vi "Save Distances.vi"(10 "Cluster":T1, 11 "Process":bool) -> ()   [LabVIEW 2016]
uses:
  <vilib>/Utility/config.llb/Write Key (Double).vi
  <vilib>/Utility/config.llb/NI_LVConfig.lvlib
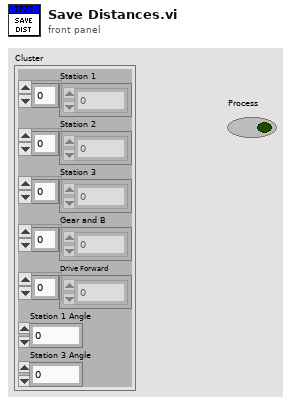
[diagram p1: front panel]
types:
  T1 = cluster{"Station 1":dbl[], "Station 2":dbl[], "Station 3":dbl[], "Gear and B":dbl[], "Drive Forward":dbl[], "Station 1 Angle":dbl, "Station 3 Angle":dbl}
  T2 = typedef "NI_LVConfig.lvlib/Config Data RefNum.ctl" = refnum<k1>
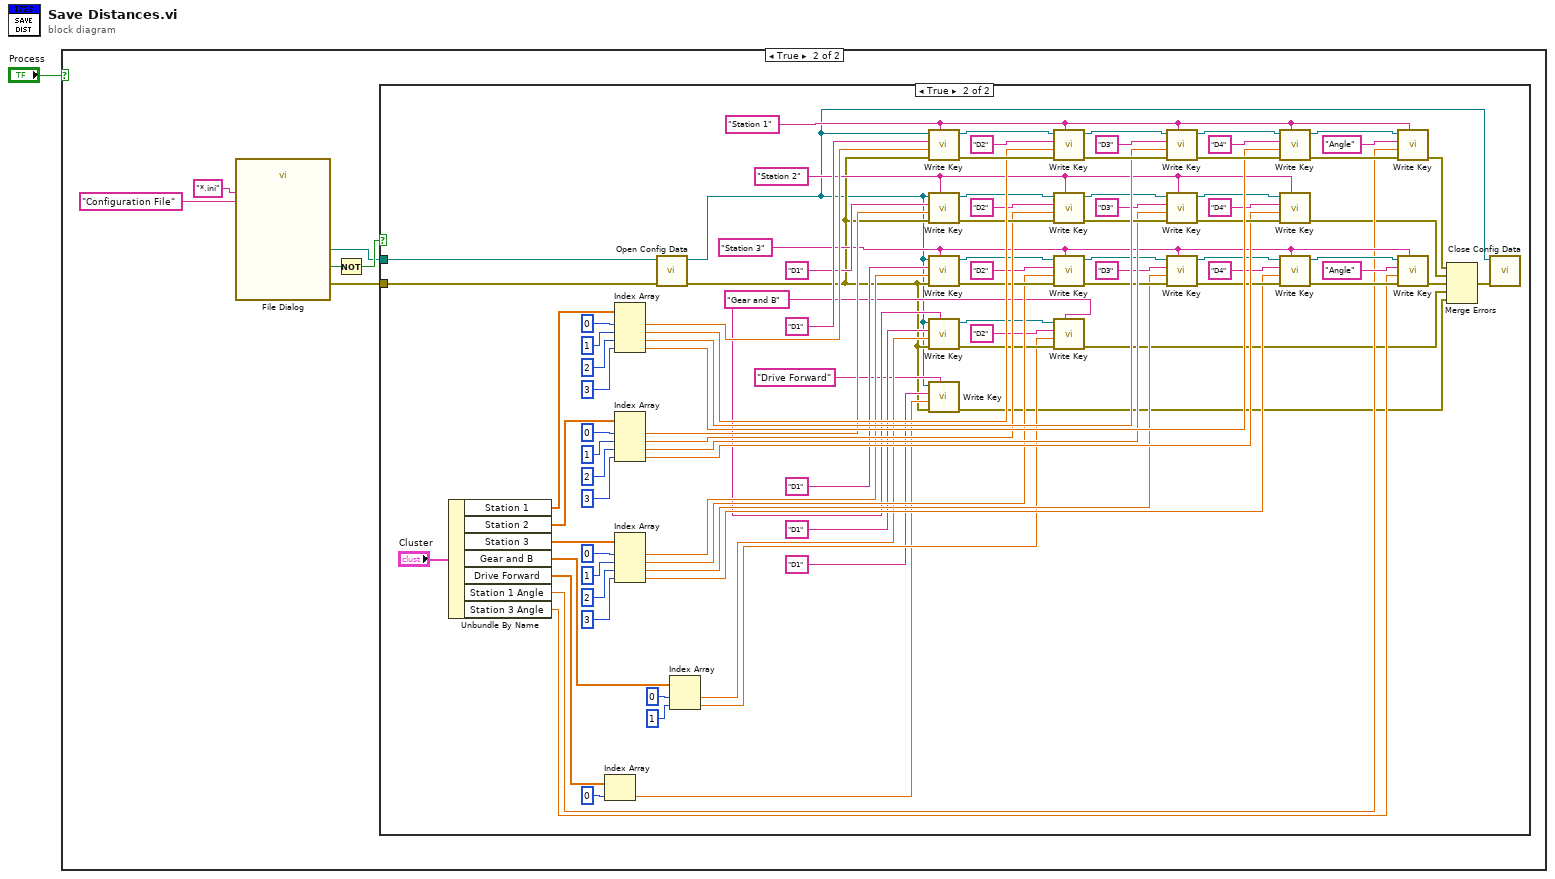
[diagram p0: block diagram]
diagram:
  n1 = case shown="True" "Process" {
    frame False {
    }
    frame True {
      n2 = call "File Dialog"("pattern (all files)"="*.ini", "pattern label"="Configuration File") -> ("selected path"=w5:path, "cancelled"=w7:bool, "error out"=w4:errorcluster)  [unwired: 10 in, 1 out]
      n3 = Not(x=w7) -> (.not. x?=w6:bool)
      n4 = case shown="True" w6 {
        tunnel: w5 -> [_ w100]
        tunnel: w4 -> [_ w99]
        frame False {
        }
        frame True {
          w31 = "Gear and B" ("section")
          w42 = "Station 3" ("section")
          w65 = "Station 2" ("section")
          w76 = "Station 1" ("section")
          n5 = Unbundle By Name("Cluster") -> ("Station 1"=w91:dbl[], "Station 2"=w60:dbl[], "Station 3"=w37:dbl[], "Gear and B"=w24:dbl[], "Drive Forward"=w17:dbl[], "Station 1 Angle"=w19:dbl, "Station 3 Angle"=w32:dbl)
          n6 = Index Array(array=w17, index=0) -> (element=w16:dbl)
          n7 = Index Array(array=w91, index #1=0 ("index"), index #2=1 ("index"), index #3=2 ("index"), index #4=3 ("index")) -> (element #1=w83:dbl, element #2=w82:dbl, element #3=w81:dbl, element #4=w80:dbl)
          n8 = Index Array(array=w60, index #1=0 ("index"), index #2=1 ("index"), index #3=2 ("index"), index #4=3 ("index")) -> (element #1=w59:dbl, element #2=w58:dbl, element #3=w57:dbl, element #4=w56:dbl)
          n9 = Index Array(array=w37, index #1=0 ("index"), index #2=1 ("index"), index #3=2 ("index"), index #4=3 ("index")) -> (element #1=w36:dbl, element #2=w35:dbl, element #3=w34:dbl, element #4=w33:dbl)
          n10 = call <vilib>:"Open Config Data.vi"("error in (no error)"=w99, "configuration file path"=w100) -> ("error out"=w15:errorcluster, "refnum"=w8:T2)  [unwired: 7 in, 1 out]
          n11 = Index Array(array=w24, index #1=0 ("index"), index #2=1 ("index")) -> (element #1=w23:dbl, element #2=w22:dbl)
          n12 = call-poly <vilib>:"Write Key.vi"("section"=w76, "error in (no error)"=w15, "value"=w83, "key"="D1", "refnum"=w8) -> ("error out"=w98:errorcluster, "refnum out"=w93:T2)  [unwired: 4 in, 1 out]
          n13 = call-poly <vilib>:"Write Key.vi"("section"=w65, "error in (no error)"=w15, "value"=w59, "key"="D1", "refnum"=w8) -> ("error out"=w75:errorcluster, "refnum out"=w70:T2)  [unwired: 4 in, 1 out]
          n14 = call-poly <vilib>:"Write Key.vi"("section"=w42, "error in (no error)"=w15, "value"=w36, "key"="D1", "refnum"=w8) -> ("error out"=w55:errorcluster, "refnum out"=w50:T2)  [unwired: 4 in, 1 out]
          n15 = call-poly <vilib>:"Write Key.vi"("section"=w31, "error in (no error)"=w15, "value"=w23, "key"="D1", "refnum"=w8) -> ("error out"=w27:errorcluster, "refnum out"=w30:T2)  [unwired: 4 in, 1 out]
          n16 = call-poly <vilib>:"Write Key.vi"("section"="Drive Forward", "error in (no error)"=w15, "value"=w16, "key"="D1", "refnum"=w8) -> ("error out"=w10:errorcluster)  [unwired: 4 in, 2 out]
          n17 = call-poly <vilib>:"Write Key.vi"("section"=w76, "error in (no error)"=w98, "value"=w82, "key"="D2", "refnum"=w93) -> ("error out"=w97:errorcluster, "refnum out"=w92:T2)  [unwired: 4 in, 1 out]
          n18 = call-poly <vilib>:"Write Key.vi"("section"=w65, "error in (no error)"=w75, "value"=w58, "key"="D2", "refnum"=w70) -> ("error out"=w74:errorcluster, "refnum out"=w69:T2)  [unwired: 4 in, 1 out]
          n19 = call-poly <vilib>:"Write Key.vi"("section"=w42, "error in (no error)"=w55, "value"=w35, "key"="D2", "refnum"=w50) -> ("error out"=w54:errorcluster, "refnum out"=w49:T2)  [unwired: 4 in, 1 out]
          n20 = call-poly <vilib>:"Write Key.vi"("section"=w31, "error in (no error)"=w27, "value"=w22, "key"="D2", "refnum"=w30) -> ("error out"=w11:errorcluster)  [unwired: 4 in, 2 out]
          n21 = call-poly <vilib>:"Write Key.vi"("section"=w76, "error in (no error)"=w97, "value"=w81, "key"="D3", "refnum"=w92) -> ("error out"=w85:errorcluster, "refnum out"=w84:T2)  [unwired: 4 in, 1 out]
          n22 = call-poly <vilib>:"Write Key.vi"("section"=w65, "error in (no error)"=w74, "value"=w57, "key"="D3", "refnum"=w69) -> ("error out"=w67:errorcluster, "refnum out"=w66:T2)  [unwired: 4 in, 1 out]
          n23 = call-poly <vilib>:"Write Key.vi"("section"=w42, "error in (no error)"=w54, "value"=w34, "key"="D3", "refnum"=w49) -> ("error out"=w47:errorcluster, "refnum out"=w46:T2)  [unwired: 4 in, 1 out]
          n24 = call-poly <vilib>:"Write Key.vi"("section"=w76, "error in (no error)"=w85, "value"=w80, "key"="D4", "refnum"=w84) -> ("error out"=w78:errorcluster, "refnum out"=w77:T2)  [unwired: 4 in, 1 out]
          n25 = call-poly <vilib>:"Write Key.vi"("section"=w65, "error in (no error)"=w67, "value"=w56, "key"="D4", "refnum"=w66) -> ("error out"=w13:errorcluster)  [unwired: 4 in, 2 out]
          n26 = call-poly <vilib>:"Write Key.vi"("section"=w42, "error in (no error)"=w47, "value"=w33, "key"="D4", "refnum"=w46) -> ("error out"=w44:errorcluster, "refnum out"=w43:T2)  [unwired: 4 in, 1 out]
          n27 = call-poly <vilib>:"Write Key.vi"("section"=w76, "error in (no error)"=w78, "value"=w19, "key"="Angle", "refnum"=w77) -> ("error out"=w14:errorcluster)  [unwired: 4 in, 2 out]
          n28 = call-poly <vilib>:"Write Key.vi"("section"=w42, "error in (no error)"=w44, "value"=w32, "key"="Angle", "refnum"=w43) -> ("error out"=w12:errorcluster)  [unwired: 4 in, 2 out]
          n29 = Merge Errors(w14, w13, w12, w11, w10) -> (w9:errorcluster)
          n30 = call <vilib>:"Close Config Data.vi"("error in (no error)"=w9, "refnum"=w8) -> ()  [unwired: 8 in, 2 out]
        }
      }
    }
  }
